vi "Main.Start.vi"(11 "State Variables in":T1 {"Protocol App"."MonitorTool.Network"."Name" format="%.0x"; "Protocol App"."Data"."Timing.Refs"."Data Reference" format="%.0x"; "Protocol App"."Data"."Network"."Name" format="%.0x"; "Protocol App"."Data"."IncomingRefs"."Data Reference" format="%.0x"; "Protocol App"."Data"."OutgoingRefs"."Data Reference" format="%.0x"; "Protocol App"."XNET Settings"."Termination" items=["Off", "On"]}) -> (0 "error out":errorcluster, 3 "State Variables out":T1 {"Protocol App"."MonitorTool.Network"."Name" format="%.0x"; "Protocol App"."Data"."Timing.Refs"."Data Reference" format="%.0x"; "Protocol App"."Data"."Network"."Name" format="%.0x"; "Protocol App"."Data"."IncomingRefs"."Data Reference" format="%.0x"; "Protocol App"."Data"."OutgoingRefs"."Data Reference" format="%.0x"; "Protocol App"."XNET Settings"."Termination" items=["Off", "On"]})   [LabVIEW 2015, in "J1939 Addon Engine.lvlib"]
uses:
  J1939 Addon Engine.lvlib
  Types/Main.State Variables.ctl
  <vilib>/NI/NIVS Inline Async API/_VS Inline Async API/VS Inline Async API/VS Inline Async API.lvclass
  Types/Main.Settings.ctl
  Types/Protocol.App Settings.ctl
  Shared/Types/XNET Settings.ctl
  Types/Protocol.XNET Refs.ctl
  <vilib>/NI Veristand/Custom Device API/Block Data Reference.ctl
  <vilib>/NI Veristand/Custom Device API/Data Reference.ctl
  Shared/Types/Monitor Settings.ctl
  Types/Engine.DTC Settings.ctl
  Shared/Types/Compiled Simulated Settings.ctl
  Types/Engine.DTC FIFOs.ctl
  <vilib>/xnet/xnet.llb/XNET Control Scope.ctl
  <resource>/objmgr/xnet.rc
  <vilib>/NI VeriStand/Custom Device API/Custom Device API.lvlib
  Shared/J1939 Addon Shared.lvlib
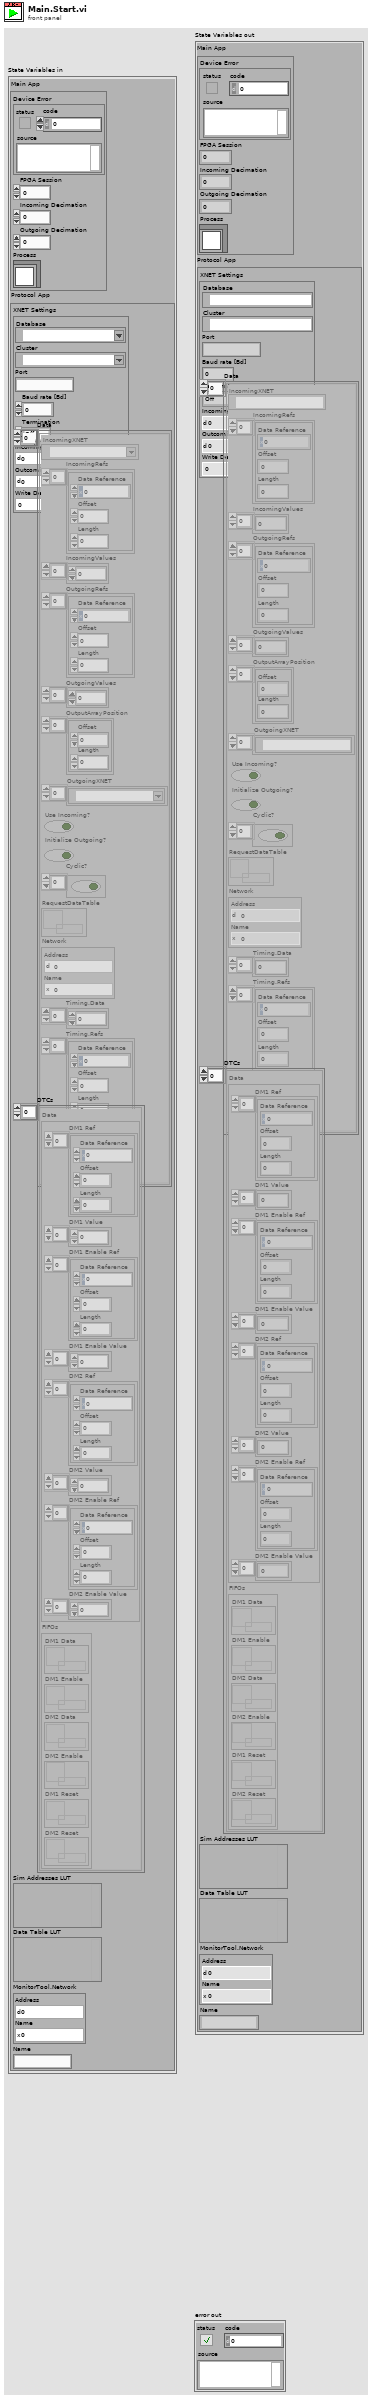
[diagram p1: front panel]
types:
  T1 = typedef "J1939 Addon Engine.lvlib/Main.State Variables.ctl" = cluster{"Main App":T2, "Protocol App":T3}
  T2 = typedef "J1939 Addon Engine.lvlib/Main.Settings.ctl" = cluster{"Device Error":errorcluster, "FPGA Session":u32, "Incoming Decimation":u32, "Outgoing Decimation":u32, "Process":refnum<class "VS Inline Async API.lvclass">}
  T3 = typedef "J1939 Addon Engine.lvlib/Protocol.App Settings.ctl" = cluster{"XNET Settings":T4, "Data":T5[], "DTCs":T9[], "Sim Addresses LUT":variant, "Data Table LUT":variant, "MonitorTool.Network":T8, "Name":string}
  T4 = typedef "J1939 Addon Shared.lvlib/XNET Settings.ctl" = cluster{"Database":refnum<k21>, "Cluster":refnum<k21>, "Port":string, "Baud rate [Bd]":u32, "Termination":u32, "Incoming Rate":u32, "Outcoming Rate":u32, "Write Decimation":u32}
  T5 = typedef "J1939 Addon Engine.lvlib/Protocol.XNET Refs.ctl" = cluster{"IncomingXNET":refnum<k21>, "IncomingRefs":T6[], "IncomingValues":dbl[], "OutgoingRefs":T6[], "OutgoingValues":dbl[], "OutputArrayPosition":cluster{"Offset":u32, "Length":u32}[], "OutgoingXNET":refnum<k21>[], "Use Incoming?":bool, "Initialize Outgoing?":bool, "Cyclic?":bool[], "RequestDataTable":refnum<k33>, "Network":T8, "Timing.Data":dbl[], "Timing.Refs":T6[], "Timing.Index":i32[], "Timing.Use":bool}
  T6 = typedef "Custom Device API.lvlib/Block Data Reference.ctl" = cluster{"Data Reference":T7, "Offset":u64, "Length":u64}
  T7 = typedef "Custom Device API.lvlib/Data Reference.ctl" = i32
  T8 = typedef "J1939 Addon Shared.lvlib/Monitor Settings.ctl" = cluster{"Address":u8, "Name":u64}
  T9 = typedef "J1939 Addon Engine.lvlib/Engine.DTC Settings.ctl" = cluster{"Data":T10, "FIFOs":T11}
  T10 = typedef "J1939 Addon Shared.lvlib/Compiled Simulated Settings.ctl" = cluster{"DM1 Ref":T6[], "DM1 Value":dbl[], "DM1 Enable Ref":T6[], "DM1 Enable Value":dbl[], "DM2 Ref":T6[], "DM2 Value":dbl[], "DM2 Enable Ref":T6[], "DM2 Enable Value":dbl[]}
  T11 = typedef "J1939 Addon Engine.lvlib/Engine.DTC FIFOs.ctl" = cluster{"DM1 Data":refnum<k33>, "DM1 Enable":refnum<k33>, "DM2 Data":refnum<k33>, "DM2 Enable":refnum<k33>, "DM1 Reset":refnum<k33>, "DM2 Reset":refnum<k33>}
  T12 = typedef "XNET Control Scope.ctl" = u32
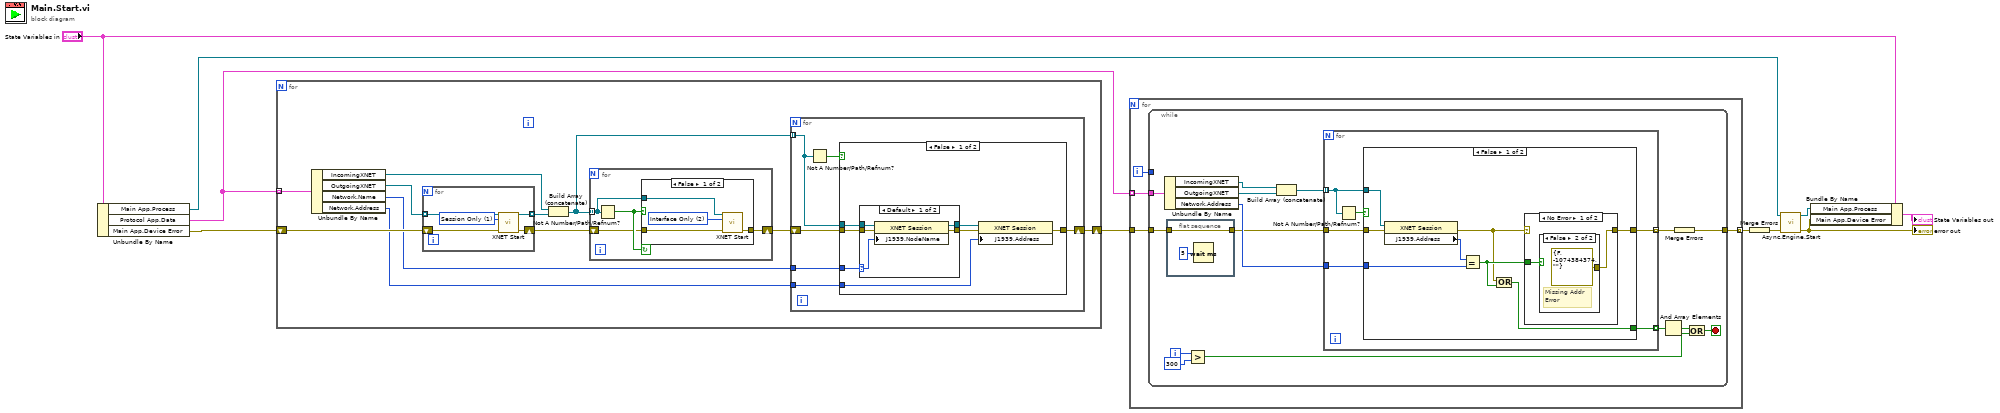
[diagram p0: block diagram]
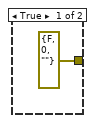
[diagram p2: hidden frame]
diagram:
  n1 = Unbundle By Name("State Variables in") -> ("Main App.Process"=w2:refnum<class "VS Inline Async API.lvclass">, "Protocol App.Data"=w5:T5[], "Main App.Device Error"=w10:errorcluster)
  n2 = for {
    shift-right: [w14] -> w7
    shift-left: w10 -> [w20]
    tunnel: w5 -> [w19] mode=indexing
    n3 = Unbundle By Name(w19) -> ("IncomingXNET"=w18:refnum<k21>, "OutgoingXNET"=w21:refnum<k21>[], "Network.Name"=w13:u64, "Network.Address"=w12:u8)
    n4 = for {
      tunnel: w21 -> [w55] mode=indexing
      shift-right: [w53] -> w16
      shift-left: w20 -> [w54]
      tunnel: [w52] -> w17 mode=indexing
      w56 = T12 1 items=["Normal", "Session Only", "Interface Only", "Session Only Blocking"] ("scope (normal)")
      n5 = call <vilib>:"XNET Start.vi"("session in"=w55, "scope (normal)"=w56, "error in (no error)"=w54) -> ("session out"=w52:refnum<k21>, "error out"=w53:errorcluster)  [unwired: 11 in]
    }
    n6 = Build Array (concatenate)(w18, w17) -> (w11:refnum<k21>[])
    n7 = for {
      tunnel: w11 -> [w44] mode=indexing
      shift-right: [w43] -> w15
      shift-left: w16 -> [w45]
      stop <- w46 continue-if-true
      n8 = Not A Number/Path/Refnum?(number/path/refnum=w44) -> (NaN/Path/Refnum?=w46:bool)
      n9 = case shown="False" w46 {
        tunnel: w45 -> [w48 w51]
        tunnel: w44 -> [w49 _]
        tunnel: [w47 w51] -> w43
        frame False {
          w50 = T12 2 items=["Normal", "Session Only", "Interface Only", "Session Only Blocking"] ("scope (normal)")
          n10 = call <vilib>:"XNET Start.vi"("session in"=w49, "scope (normal)"=w50, "error in (no error)"=w48) -> ("error out"=w47:errorcluster)  [unwired: 11 in, 1 out]
        }
        frame True {
        }
      }
    }
    n11 = for {
      tunnel: w11 -> [w25] mode=indexing
      shift-right: [w24] -> w14
      shift-left: w15 -> [w26]
      tunnel: w13 -> [w23]
      tunnel: w12 -> [w22]
      n12 = Not A Number/Path/Refnum?(number/path/refnum=w25) -> (NaN/Path/Refnum?=w27:bool)
      n13 = case shown="False" w27 {
        tunnel: w26 -> [w33 w42]
        tunnel: w25 -> [w34 _]
        tunnel: [w32 w42] -> w24
        tunnel: w23 -> [w29 _]
        tunnel: w22 -> [w30 _]
        frame False {
          n14 = case shown="Default" w29 {
            selector: w29 -> [w37 _]
            tunnel: w34 -> [w39 w40]
            tunnel: w33 -> [w38 w41]
            tunnel: [w36 w41] -> w31
            tunnel: [w35 w40] -> w28
            frame Default {
              n15 = property class="XNET Session"(reference=w39, error in=w38, "J1939.NodeName"=w37) -> (reference out=w35:refnum<k21>, error out=w36:errorcluster)
            }
            frame 0 {
            }
          }
          n16 = property class="XNET Session"(reference=w28, error in=w31, "J1939.Address"=w30) -> (error out=w32:errorcluster)  [unwired: 1 out]
        }
        frame True {
        }
      }
    }
  }
  n17 = for {
    tunnel: w5 -> [w60] mode=indexing
    tunnel: w7 -> [w59]
    tunnel: [w58] -> w6 mode=indexing
    i -> [w57]
    n18 = while {
      tunnel: w60 -> [w73]
      tunnel: w59 -> [w67]
      tunnel: [w70] -> w58
      tunnel: w57 -> [_]
      i -> [w65]
      stop <- w61 stop-if-true
      n19 = Unbundle By Name(w73) -> ("IncomingXNET"=w75:refnum<k21>, "OutgoingXNET"=w74:refnum<k21>[], "Network.Address"=w69:u8)
      n20 = flat-sequence {
        tunnel: [w77] -> w68
        tunnel: w67 -> [w77]
        frame #0 {
          n21 = Wait (ms)(milliseconds to wait=u32 5) -> ()  [unwired: 1 out]
        }
      }
      n22 = Greater?(x=w65, y=300) -> (0:w62:bool)
      n23 = Build Array (concatenate)(w75, w74) -> (w71:refnum<k21>[])
      n24 = for {
        tunnel: w68 -> [w83]
        tunnel: [w82] -> w72 mode=indexing
        tunnel: w71 -> [w81] mode=indexing
        tunnel: w69 -> [w79]
        tunnel: [w78] -> w64 mode=indexing
        n25 = Not A Number/Path/Refnum?(number/path/refnum=w81) -> (NaN/Path/Refnum?=w80:bool)
        n26 = case shown="False" w80 {
          selector: w80 -> [_ w97]
          tunnel: w83 -> [w89 w98]
          tunnel: [w88 w98] -> w82
          tunnel: w81 -> [w86 _]
          tunnel: w79 -> [w87 _]
          tunnel: [w84 w97] -> w78
          frame False {
            n27 = property class="XNET Session"(reference=w86, error in=w89) -> (error out=w90:errorcluster, "J1939.Address"=w85:u8)  [unwired: 1 out]
            n28 = Equal?(x=w85, y=w87) -> (x = y?=w91:bool)
            n29 = Compound Arithmetic op=OR(w90, w91) -> (w84:bool)
            n30 = case shown="No Error" w90 {
              selector: w90 -> [_ w96]
              tunnel: w91 -> [w93 _]
              tunnel: [w92 w96] -> w88
              frame No Error {
                n31 = case shown="False" w93 {
                  tunnel: [errorcluster {"status"=FALSE, "code"=0, "source"=""} ("error out") errorcluster {"status"=FALSE, "code"=-1074384374, "source"=""} ("error out")] -> w92
                  frame True {
                  }
                  frame False {
                    # "Missing Addr\nError"
                  }
                }
              }
              frame Error {
              }
            }
          }
          frame True {
          }
        }
      }
      n32 = And Array Elements(Boolean array=w64) -> (logical AND=w63:bool)
      n33 = Merge Errors(w72) -> (w70:errorcluster)
      n34 = Compound Arithmetic op=OR(w63, w62) -> (w61:bool)
    }
  }
  n35 = Merge Errors(w6) -> (w4:errorcluster)
  n36 = call <vilib>:"Async.Engine.Start.vi"("error in (no error)"=w4, "VS Inline Async API in"=w2) -> ("error out"=w3:errorcluster, "VS Inline Async API out"=w1:refnum<class "VS Inline Async API.lvclass">)  [unwired: 8 in]
  "error out" <- w3
  n37 = Bundle By Name(cluster="State Variables in", "Main App.Process"=w1, "Main App.Device Error"=w3) -> (→"State Variables out":T1)
